vi "scope fgen pxi test.vi"() -> ()   [LabVIEW 2023]
uses:
  Scope/Scope PXI/Base CFG/Scope PXI Base CFG.lvclass
  FGen/FGen PXI/FGen PXI Std Waveform CFG/FGen PXI Std Waveform CFG.lvclass
  <vilib>/Waveform/WDTOps.llb/WDT Number of Waveform Samples DBL.vi
  Measure and Stimulus Subsystems/Measure and Stimulus Subsystems.lvclass
  Scope/Virtual Scopes/Virt Waveform Reader/Virt Waveform Reader.lvclass
  Scope/Virtual Scopes/Virt Voltage Reader/Virt Voltage Reader.lvclass
  FGen/Virtual FGens/Virt Voltage Generator/Virt Voltage Generator.lvclass
panel:
  in  "DC Gen [V]":dbl(knob) scale=0.0..1.0
  out "total samples fetched":i32
  out "#samples fetched":i32[](array[numeric])
  out "Iteration":i32
  in  "Stop":bool
  out "Photosensor Waveform Chart":waveform(dbl)(graph)
  out "Error Out":errorcluster
  out "Powersensor Scalar":dbl
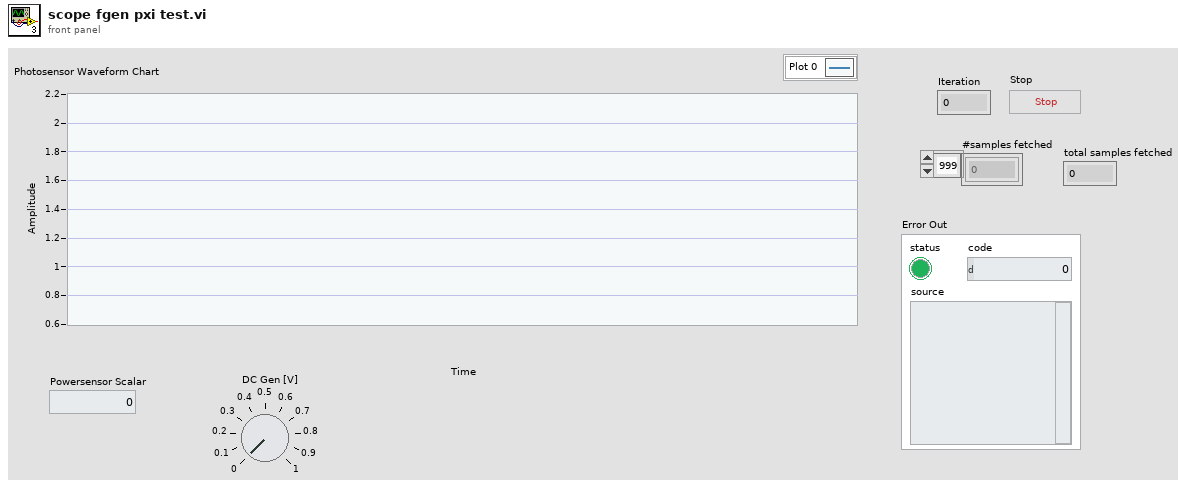
[diagram p1: front panel]
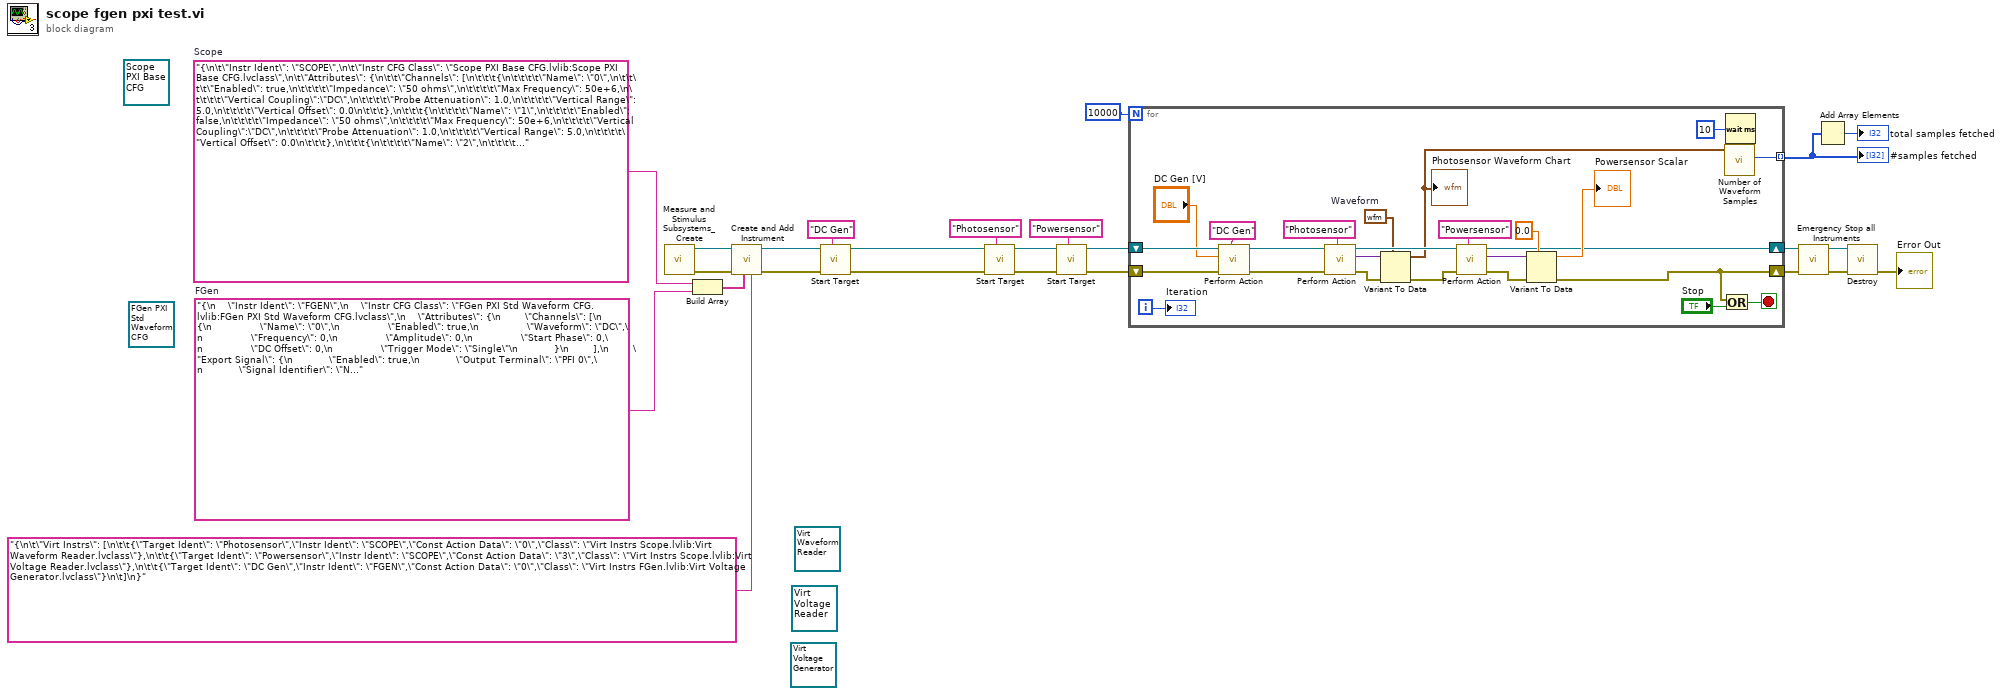
[diagram p0: block diagram]
diagram:
  (unwired) refnum<class "Virt Voltage Generator.lvclass"> refnum ("Virt Instrs FGen.lvlib:Virt Voltage Generator.lvclass")
  (unwired) refnum<class "Virt Voltage Reader.lvclass"> refnum ("Virt Instrs Scope.lvlib:Virt Voltage Reader.lvclass")
  (unwired) refnum<class "Virt Waveform Reader.lvclass"> refnum ("Virt Instrs Scope.lvlib:Virt Waveform Reader.lvclass")
  (unwired) refnum<class "FGen PXI Std Waveform CFG.lvclass"> refnum ("FGen PXI Std Waveform CFG.lvlib:FGen PXI Std Waveform CFG.lvclass")
  (unwired) refnum<class "Scope PXI Base CFG.lvclass"> refnum ("Scope PXI Base CFG.lvlib:Scope PXI Base CFG.lvclass")
  w5 = "{\n    \"Instr Ident\": \"FGEN\",\n    \"Instr CFG Class\": \"FGen PXI Std Waveform CFG.lvlib:FGen PXI Std Waveform CFG.lvclass\",\n    \"Attributes\": {\n        \"Channels\": [\n            {\n                \"Name\": \"0\",\n                \"Enabled\": true,\n                \"Waveform\": \"DC\",\n                \"Frequency\": 0,\n                \"Amplitude\": 0,\n                \"Start Phase\": 0,\n                \"DC Offset\": 0,\n                \"Trigger Mode\": \"Single\"\n            }\n        ],\n        \"Export Signal\": {\n            \"Enabled\": true,\n            \"Output Terminal\": \"PFI 0\",\n            \"Signal Identifier\": \"None\",\n            \"Signal\": \"Start Trigger\"\n        },\n        \"Output\": {\n            \"Idle\": {\n                \"Idle Behavior\": \"Jump To Value\",\n                \"Idle Value\": 0\n            }\n        }\n    }\n}"  # FGen
  w13 = "{\n\t\"Instr Ident\": \"SCOPE\",\n\t\"Instr CFG Class\": \"Scope PXI Base CFG.lvlib:Scope PXI Base CFG.lvclass\",\n\t\"Attributes\": {\n\t\t\"Channels\": [\n\t\t\t{\n\t\t\t\t\"Name\": \"0\",\n\t\t\t\t\"Enabled\": true,\n\t\t\t\t\"Impedance\": \"50 ohms\",\n\t\t\t\t\"Max Frequency\": 50e+6,\n\t\t\t\t\"Vertical Coupling\":\"DC\",\n\t\t\t\t\"Probe Attenuation\": 1.0,\n\t\t\t\t\"Vertical Range\": 5.0,\n\t\t\t\t\"Vertical Offset\": 0.0\n\t\t\t},\n\t\t\t{\n\t\t\t\t\"Name\": \"1\",\n\t\t\t\t\"Enabled\": false,\n\t\t\t\t\"Impedance\": \"50 ohms\",\n\t\t\t\t\"Max Frequency\": 50e+6,\n\t\t\t\t\"Vertical Coupling\":\"DC\",\n\t\t\t\t\"Probe Attenuation\": 1.0,\n\t\t\t\t\"Vertical Range\": 5.0,\n\t\t\t\t\"Vertical Offset\": 0.0\n\t\t\t},\n\t\t\t{\n\t\t\t\t\"Name\": \"2\",\n\t\t\t\t\"Enabled\": false,\n\t\t\t\t\"Impedance\": \"50 ohms\",\n\t\t\t\t\"Max Frequency\": 50e+6,\n\t\t\t\t\"Vertical Coupling\":\"DC\",\n\t\t\t\t\"Probe Attenuation\": 1.0,\n\t\t\t\t\"Vertical Range\": 5.0,\n\t\t\t\t\"Vertical Offset\": 0.0\n\t\t\t},\n\t\t\t{\n\t\t\t\t\"Name\": \"3\",\n\t\t\t\t\"Enabled\": true,\n\t\t\t\t\"Impedance\": \"50 ohms\",\n\t\t\t\t\"Max Frequency\": 50e+6,\n\t\t\t\t\"Vertical Coupling\":\"DC\",\n\t\t\t\t\"Probe Attenuation\": 1.0,\n\t\t\t\t\"Vertical Range\": 1.4,\n\t\t\t\t\"Vertical Offset\": 0.0\n\t\t\t},\n\t\t\t{\n\t\t\t\t\"Name\": \"4\",\n\t\t\t\t\"Enabled\": false,\n\t\t\t\t\"Impedance\": \"50 ohms\",\n\t\t\t\t\"Max Frequency\": 50e+6,\n\t\t\t\t\"Vertical Coupling\":\"DC\",\n\t\t\t\t\"Probe Attenuation\": 1.0,\n\t\t\t\t\"Vertical Range\": 5.0,\n\t\t\t\t\"Vertical Offset\": 0.0\n\t\t\t},\n\t\t\t{\n\t\t\t\t\"Name\": \"5\",\n\t\t\t\t\"Enabled\": false,\n\t\t\t\t\"Impedance\": \"50 ohms\",\n\t\t\t\t\"Max Frequency\": 50e+6,\n\t\t\t\t\"Vertical Coupling\":\"DC\",\n\t\t\t\t\"Probe Attenuation\": 1.0,\n\t\t\t\t\"Vertical Range\": 5.0,\n\t\t\t\t\"Vertical Offset\": 0.0\n\t\t\t},\n\t\t\t{\n\t\t\t\t\"Name\": \"6\",\n\t\t\t\t\"Enabled\": false,\n\t\t\t\t\"Impedance\": \"50 ohms\",\n\t\t\t\t\"Max Frequency\": 50e+6,\n\t\t\t\t\"Vertical Coupling\":\"DC\",\n\t\t\t\t\"Probe Attenuation\": 1.0,\n\t\t\t\t\"Vertical Range\": 5.0,\n\t\t\t\t\"Vertical Offset\": 0.0\n\t\t\t},\n\t\t\t{\n\t\t\t\t\"Name\": \"7\",\n\t\t\t\t\"Enabled\": false,\n\t\t\t\t\"Impedance\": \"50 ohms\",\n\t\t\t\t\"Max Frequency\": 50e+6,\n\t\t\t\t\"Vertical Coupling\":\"DC\",\n\t\t\t\t\"Probe Attenuation\": 1.0,\n\t\t\t\t\"Vertical Range\": 5.0,\n\t\t\t\t\"Vertical Offset\": 0.0\n\t\t\t}\n\t\t],\n\t\t\"Horizontal\": {\n\t\t\t\"Enforce Realtime\": true,\n\t\t\t\"Number of Records\": 1,\n\t\t\t\"Min Sample Rate\": 1e+5,\n\t\t\t\"Reference Position\":10, //percent\n\t\t\t\"Min Record Length\":1e+3\n\t\t},\n\t\t\"Acquire\": {\n\t\t\t\"Type\": \"Normal\",\n\t\t\t\"NumSamples\": 1e+4,\n  \t\"Fetch Relative To\": \"Read Pointer\" \n\t\t},\n\t\t\"Export Signal\": {\n\t\t\t\"Signal Identifier\": \"None\",\n\t\t\t\"Signal\": \"None\",\n\t\t\t\"Output Terminal\": \"None\"\n\t\t},\n\t\t\"Trigger\": {\n\t\t\t\"Type\": \"Software\",\n\t\t\t\"Slope\": \"Positive\",\n\t\t\t\"Source\": \"RTSI 0\",\n\t\t\t\"Holdoff\": 0.0,\n\t\t\t\"Delay\": 0.0\n\t\t}\n\t}\n}"  # Scope
  n1 = call "Measure and Stimulus Subsystems_Create.vi"() -> ("Error Out"=w24:errorcluster, "reference out"=w25:refnum<class "Measure and Stimulus Subsystems.lvclass">)  [unwired: 10 in]
  n2 = Build Array(w13, w5) -> (w12:string[])
  n3 = call "Create and Add Instrument.vi"("Virt Instr JSON Config"="{\n\t\"Virt Instrs\": [\n\t\t{\"Target Ident\": \"Photosensor\",\"Instr Ident\": \"SCOPE\",\"Const Action Data\": \"0\",\"Class\": \"Virt Instrs Scope.lvlib:Virt Waveform Reader.lvclass\"},\n\t\t{\"Target Ident\": \"Powersensor\",\"Instr Ident\": \"SCOPE\",\"Const Action Data\": \"3\",\"Class\": \"Virt Instrs Scope.lvlib:Virt Voltage Reader.lvclass\"},\n\t\t{\"Target Ident\": \"DC Gen\",\"Instr Ident\": \"FGEN\",\"Const Action Data\": \"0\",\"Class\": \"Virt Instrs FGen.lvlib:Virt Voltage Generator.lvclass\"}\n\t]\n}", "Physical Intr Configs"=w12, "Error In"=w24, "reference in"=w25) -> ("Error Out"=w23:errorcluster, "reference out"=w3:refnum<class "Measure and Stimulus Subsystems.lvclass">)  [unwired: 6 in]
  n4 = call "Start Target.vi"("Target Ident"="DC Gen", "Error In"=w23, "reference in"=w3) -> ("Error Out"=w4:errorcluster, "reference out"=w1:refnum<class "Measure and Stimulus Subsystems.lvclass">)  [unwired: 7 in]
  n5 = call "Start Target.vi"("Target Ident"="Photosensor" ("Target Identifier"), "Error In"=w4, "reference in"=w1) -> ("Error Out"=w15:errorcluster, "reference out"=w8:refnum<class "Measure and Stimulus Subsystems.lvclass">)  [unwired: 7 in]
  n6 = call "Start Target.vi"("Target Ident"="Powersensor", "Error In"=w15, "reference in"=w8) -> ("Error Out"=w9:errorcluster, "reference out"=w7:refnum<class "Measure and Stimulus Subsystems.lvclass">)  [unwired: 7 in]
  n7 = for {
    N: 10000 -> [_]
    shift-right: [w36] -> w18
    shift-left: w9 -> [w45]
    shift-right: [w34] -> w21
    shift-left: w7 -> [w29]
    tunnel: [w31] -> w11 mode=indexing
    i -> [w33]
    stop <- w35 stop-if-true
    w42 = waveform(dbl) {"t0"=timestamp(0 s since 1904-01-01), "dt"=1.0, "Y"=[]}  # Waveform
    n8 = call "Perform Action.vi"("Target Ident"="DC Gen", "Error In"=w45, "Input"="DC Gen [V]", "reference in"=w29) -> ("Error Out"=w30:errorcluster, "reference out"=w28:refnum<class "Measure and Stimulus Subsystems.lvclass">)  [unwired: 5 in, 1 out]
    n9 = call "Perform Action.vi"("Target Ident"="Photosensor" ("Target Identifier"), "Error In"=w30, "reference in"=w28) -> ("Error Out"=w48:errorcluster, "Output"=w43:variant, "reference out"=w49:refnum<class "Measure and Stimulus Subsystems.lvclass">)  [unwired: 6 in]
    n10 = Variant To Data(error in=w48, type=w42, Variant=w43) -> (data=w32:waveform(dbl), error out=w44:errorcluster)
    "Photosensor Waveform Chart" <- w32
    n11 = call "Perform Action.vi"("Target Ident"="Powersensor" ("Target Identifier"), "Error In"=w44, "reference in"=w49) -> ("Error Out"=w46:errorcluster, "Output"=w41:variant, "reference out"=w34:refnum<class "Measure and Stimulus Subsystems.lvclass">)  [unwired: 6 in]
    n12 = Variant To Data(error in=w46, type=0.0, Variant=w41) -> (data=→"Powersensor Scalar":dbl, error out=w36:errorcluster)
    n13 = Or(x=w36, y="Stop") -> (x .or. y?=w35:bool)
    n14 = call-poly <vilib>:"Number of Waveform Samples.vi"("waveform in"=w32) -> ("number of samples"=w31:i32)  [unwired: 8 in, 2 out]
    n15 = Wait (ms)(milliseconds to wait=u32 10) -> ()  [unwired: 1 out]
    "Iteration" <- w33
  }
  "#samples fetched" <- w11
  n16 = call "Emergency Stop all Instruments.vi"("Error In"=w18, "reference in"=w21) -> ("Error Out"=w22:errorcluster, "reference out"=w20:refnum<class "Measure and Stimulus Subsystems.lvclass">)  [unwired: 8 in]
  n17 = Add Array Elements(numeric array=w11) -> (sum=→"total samples fetched":i32)
  n18 = call "Destroy.vi"("Error In"=w22, "reference in"=w20) -> ("Error Out"=→"Error Out":errorcluster)  [unwired: 8 in, 1 out]
